vi "Timer Example.vi"() -> ()   [LabVIEW 2020]
uses:
  Timer/Method/New.vi
  Timer/Method/Auto Reset.vi
  Timer/Method/Reset.vi
  Timer/Method/Wait.vi
  Timer/Method/Pause.vi
  Timer/Method/Continue.vi
  Timer/Method/Delete.vi
  Timer/Timer.lvclass
panel:
  in  "stop":bool
  in  "auto reset":bool=TRUE
  in  "continue":bool
  in  "pause":bool
  out "elapsed time(s)":dbl
  in  "error in (no error)":errorcluster
  out "error out":errorcluster
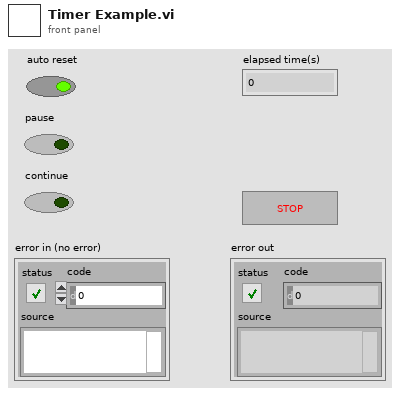
[diagram p1: front panel]
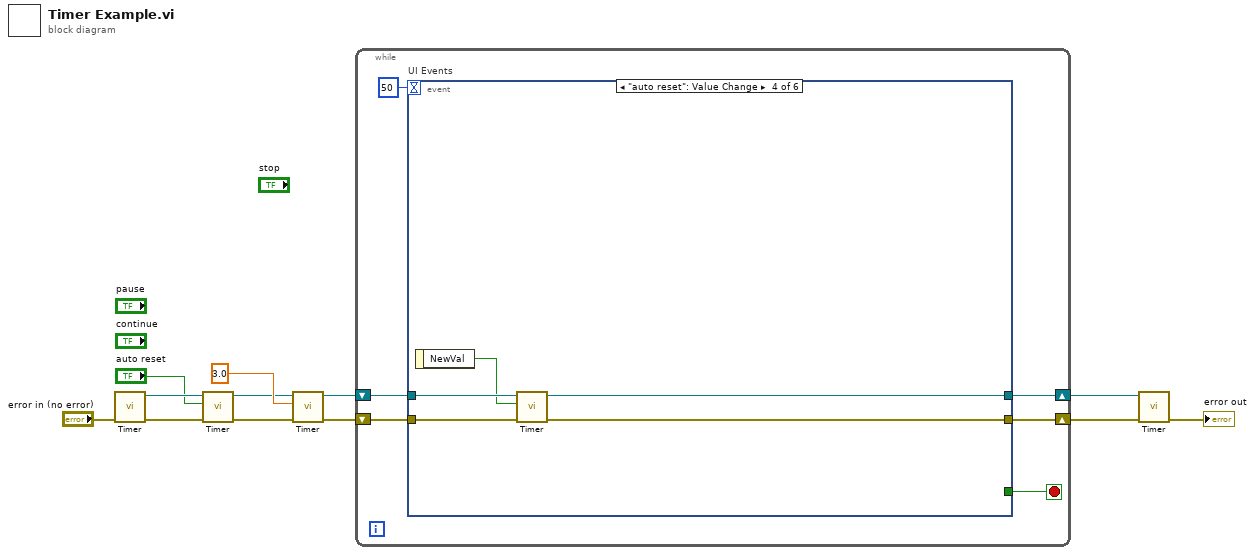
[diagram p0: block diagram]
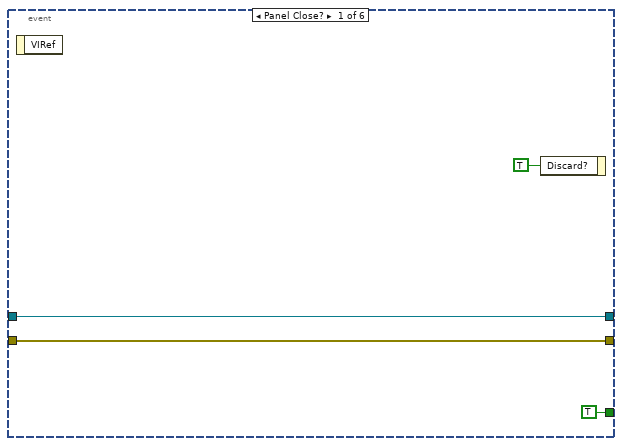
[diagram p2: hidden frame]
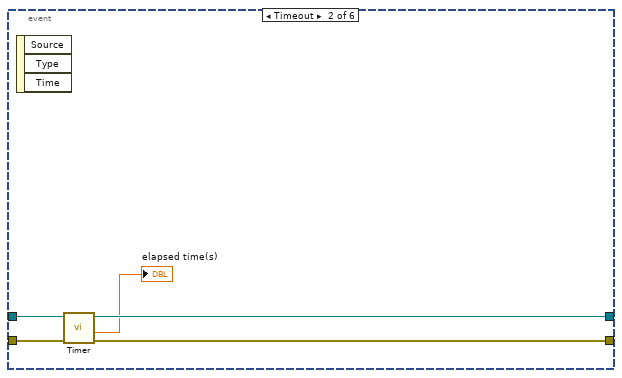
[diagram p3: hidden frame]
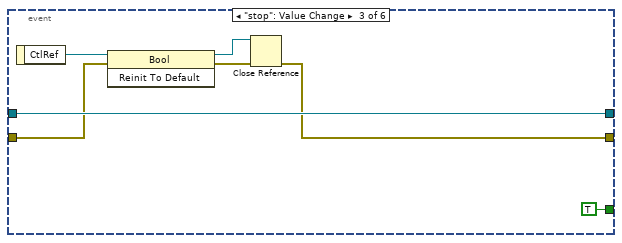
[diagram p4: hidden frame]
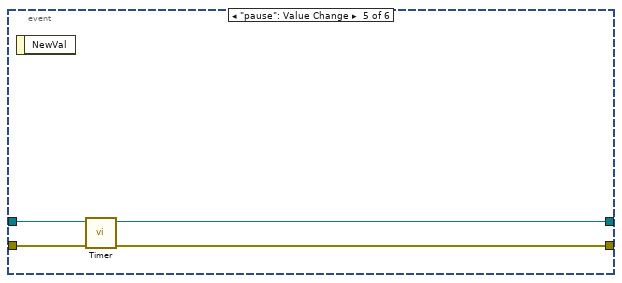
[diagram p5: hidden frame]
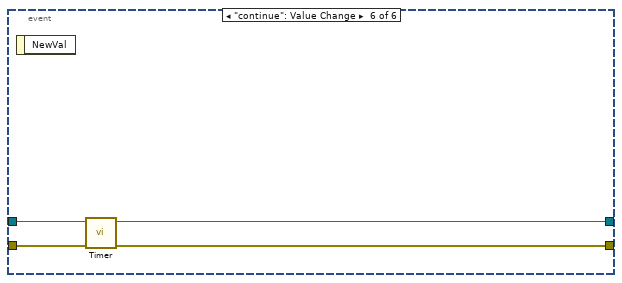
[diagram p6: hidden frame]
diagram:
  n1 = call-poly "Timer.vi"("error in (no error)"="error in (no error)") -> ("error out"=w5:errorcluster, "Timer out"=w4:refnum<class "Timer.lvclass">)  [unwired: 9 in]
  n2 = call-poly "Timer.vi"("error in (no error)"=w5, "auto reset"="auto reset", "Timer in"=w4) -> ("error out"=w1:errorcluster, "Timer out"=w2:refnum<class "Timer.lvclass">)  [unwired: 7 in]
  n3 = call-poly "Timer.vi"("error in (no error)"=w1, "target time(1s)"=3.0 ("target time(s)"), "Timer in"=w2) -> ("error out"=w7:errorcluster, "Timer out"=w8:refnum<class "Timer.lvclass">)  [unwired: 7 in]
  n4 = while {
    shift-right: [w16] -> w11
    shift-left: w7 -> [w17]
    shift-right: [w14] -> w9
    shift-left: w8 -> [w15]
    stop <- w18 stop-if-true
    n5 = event "UI Events" shown="[3] \"auto reset\": Value Change" {
      selector: _ -> [_ _ _ _ _ _]
      dyn-events: _ -> [_ _ _ _ _ _]
      timeout: 50 -> [_ _ _ _ _ _]
      tunnel: [TRUE ("stop") _ TRUE ("stop") _ _ _] -> w18
      tunnel: w17 -> [w21 w27 w31 w39 w43 w47]
      tunnel: [w21 w23 w28 w35 w40 w44] -> w16
      tunnel: w15 -> [w19 w26 w34 w38 w42 w46]
      tunnel: [w19 w25 w34 w36 w41 w45] -> w14
      event Panel Close? {
        n6 = event-data() -> ()  [unwired: 1 in, 1 out]
        n7 = event-data("Discard?"=TRUE) -> ()  [unwired: 1 in, 1 out]
      }
      event Timeout {
        n8 = event-data() -> ()  [unwired: 1 in, 3 out]
        n9 = call-poly "Timer.vi"("error in (no error)"=w27, "Timer in"=w26) -> ("error out"=w23:errorcluster, "elapsed time(s)"=→"elapsed time(s)":dbl, "Timer out"=w25:refnum<class "Timer.lvclass">)  [unwired: 6 in, 1 out]
      }
      event "stop": Value Change {
        n10 = event-data() -> ("CtlRef"=w32:refnum<vi>)  [unwired: 1 in]
        n11 = invoke class="Bool" method="Reinit To Default"(reference=w32, error in=w31) -> (reference out=w29:refnum<vi>, error out=w30:errorcluster)  [unwired: 1 in, 1 out]
        n12 = Close Reference(reference=w29, error in (no error)=w30) -> (error out=w28:errorcluster)
      }
      event "auto reset": Value Change {
        n13 = event-data() -> ("NewVal"=w37:bool)  [unwired: 1 in]
        n14 = call-poly "Timer.vi"("error in (no error)"=w39, "auto reset"=w37, "Timer in"=w38) -> ("error out"=w35:errorcluster, "Timer out"=w36:refnum<class "Timer.lvclass">)  [unwired: 7 in]
      }
      event "pause": Value Change {
        n15 = event-data() -> ()  [unwired: 1 in, 1 out]
        n16 = call-poly "Timer.vi"("error in (no error)"=w43, "Timer in"=w42) -> ("error out"=w40:errorcluster, "Timer out"=w41:refnum<class "Timer.lvclass">)  [unwired: 8 in]
      }
      event "continue": Value Change {
        n17 = event-data() -> ()  [unwired: 1 in, 1 out]
        n18 = call-poly "Timer.vi"("error in (no error)"=w47, "Timer in"=w46) -> ("error out"=w44:errorcluster, "Timer out"=w45:refnum<class "Timer.lvclass">)  [unwired: 8 in]
      }
    }
  }
  n19 = call-poly "Timer.vi"("error in (no error)"=w11, "Timer in"=w9) -> ("error out"=→"error out":errorcluster)  [unwired: 9 in]
